vi "Check Action.vi"(6 "HRS Time":dbl, 7 "Values In":dbl[](array[numeric]), 8 "error in (no error)":errorcluster, 11 "Valve in":refnum<class "MultiControl.lvclass">) -> (0 "error out":errorcluster, 2 "Actions":T1[](array[typedef]), 3 "Valve out":refnum<class "MultiControl.lvclass">, 5 "Values":dbl[](array[numeric]))   [LabVIEW 2020, in "VolatusControl.lvlib" / "MultiControl.lvclass"]
uses:
  MultiControl.lvclass
  Control Action.ctl
  MultiControl.lvclass/MultiControl.ctl
  lv-vecto/Vecto/Vecto.lvlib
  Volatus/MessageQ/MessageQ.lvclass
  VolatusControl.lvlib
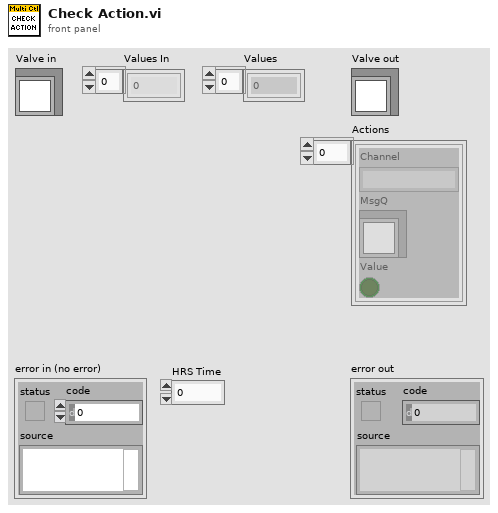
[diagram p1: front panel]
types:
  T1 = typedef "VolatusControl.lvlib/Control Action.ctl" = cluster{"Channel":string, "MsgQ":refnum<class "MessageQ.lvclass">, "Value":bool}
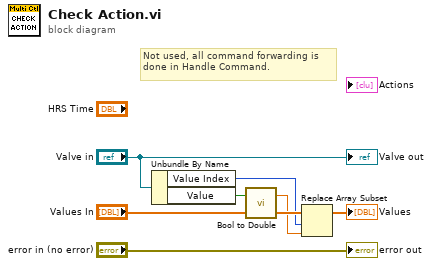
[diagram p0: block diagram]
diagram:
  # "Not used, all command forwarding is done in Handle Command."
  n1 = Unbundle By Name("Valve in") -> ("Value Index"=w2:i32, "Value"=w3:bool)
  n2 = call "Bool to Double.vi"("Bool"=w3) -> ("Double"=w1:dbl)  [unwired: 2 in]
  n3 = Replace Array Subset(array="Values In", new element=w1, index=w2) -> (→"Values":dbl[])
  "error out" <- "error in (no error)"
  "Valve out" <- "Valve in"
